vi "生成校准记录.vi"(0 "标液一":cluster{"标准值":dbl, "检测值":dbl, "原始值":dbl} caption="标液一：" {"原始值" format="%#.6f"; "检测值" format="%#.6f"; "标准值" format="%#.6f"}, 1 "校准参数":u16(ring) caption="校准参数：" items=["pH", "DO", "浊度", "电导率", "叶绿素a", "藻密度", "ORP", "COD", "DO2", "氯化物", "氨氮", "水中油"], 2 "校准方式":u16(ring) caption="校准方式：" items=["单点校准", "两点校准", "三点校准"], 3 "校准记录":refnum<vi>, 5 "标液二":cluster{"标准值":dbl, "检测值":dbl, "原始值":dbl} caption="标液二：" {"原始值" format="%#.6f"; "检测值" format="%#.6f"; "标准值" format="%#.6f"}, 7 "标液三":cluster{"标准值":dbl, "检测值":dbl, "原始值":dbl} caption="标液三：" {"原始值" format="%#.6f"; "检测值" format="%#.6f"; "标准值" format="%#.6f"}, 9 "当前温度":dbl caption="当前温度：" format="%.2f ℃", 11 "error in (no error)":errorcluster caption="错误输入（无错误）", 12 "序列号":string caption="序列号：", 13 "K":dbl=25.0 caption="电极系数：" format="%#_6f", 14 "B":dbl=25.0 caption="电极零点：" format="%#_6f") -> (4 "校准记录":string="校准记录\n---------------------------------------------\n序列号：\n温度值：\n标准值：\n检测值：\n原始值：\n校准时间：", 15 "error out":errorcluster caption="错误输出")   [LabVIEW 2022 SP3, in "斯坦道多参数.lvlib"]
uses:
  <vilib>/Utility/miscctls.llb/LVFontTypeDef.ctl
panel:
  in  "选项卡控件":enum32{"选项卡 1"}(tab)
  # "检测值"
  # "原始值"
  # "标准值"
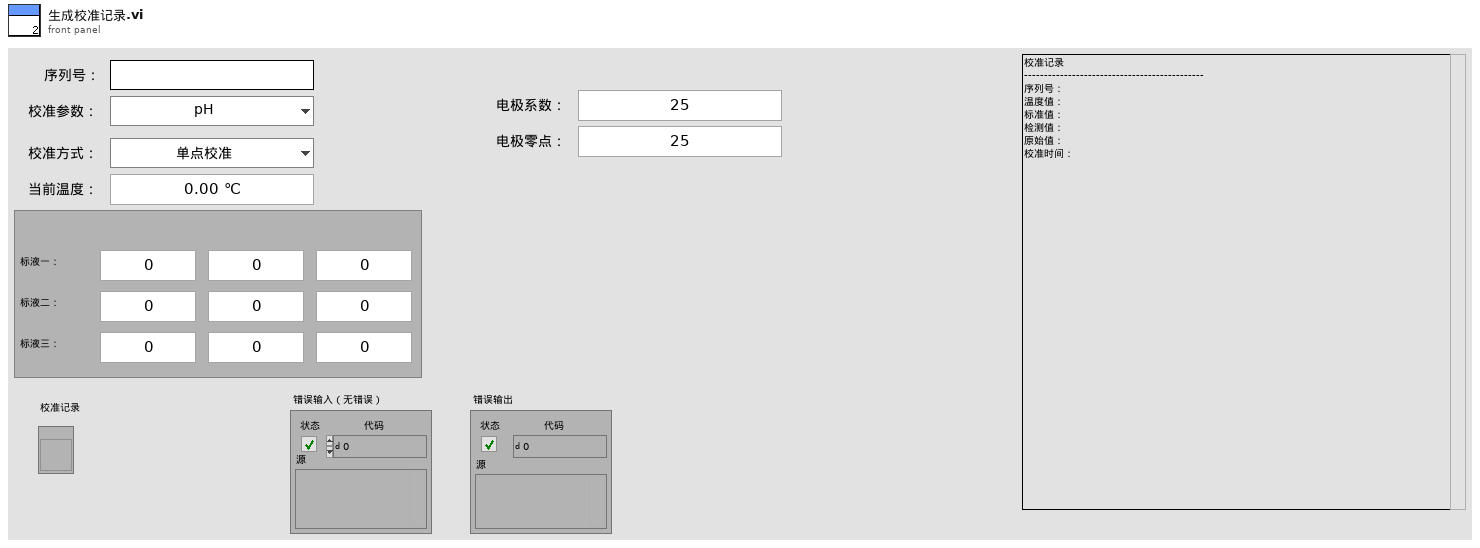
[diagram p1: front panel]
types:
  T1 = typedef "LVFontTypeDef.ctl" = cluster{"Font Name":string, "Size":u16, "Bold":bool, "Italic":bool, "Underline":bool, "Strikeout":bool, "Color":u32}
  T2 = typedef "斯坦道多参数.lvlib/探头类型.ctl" = enum16{"禹山", "国弘", "纳清", "STD"}
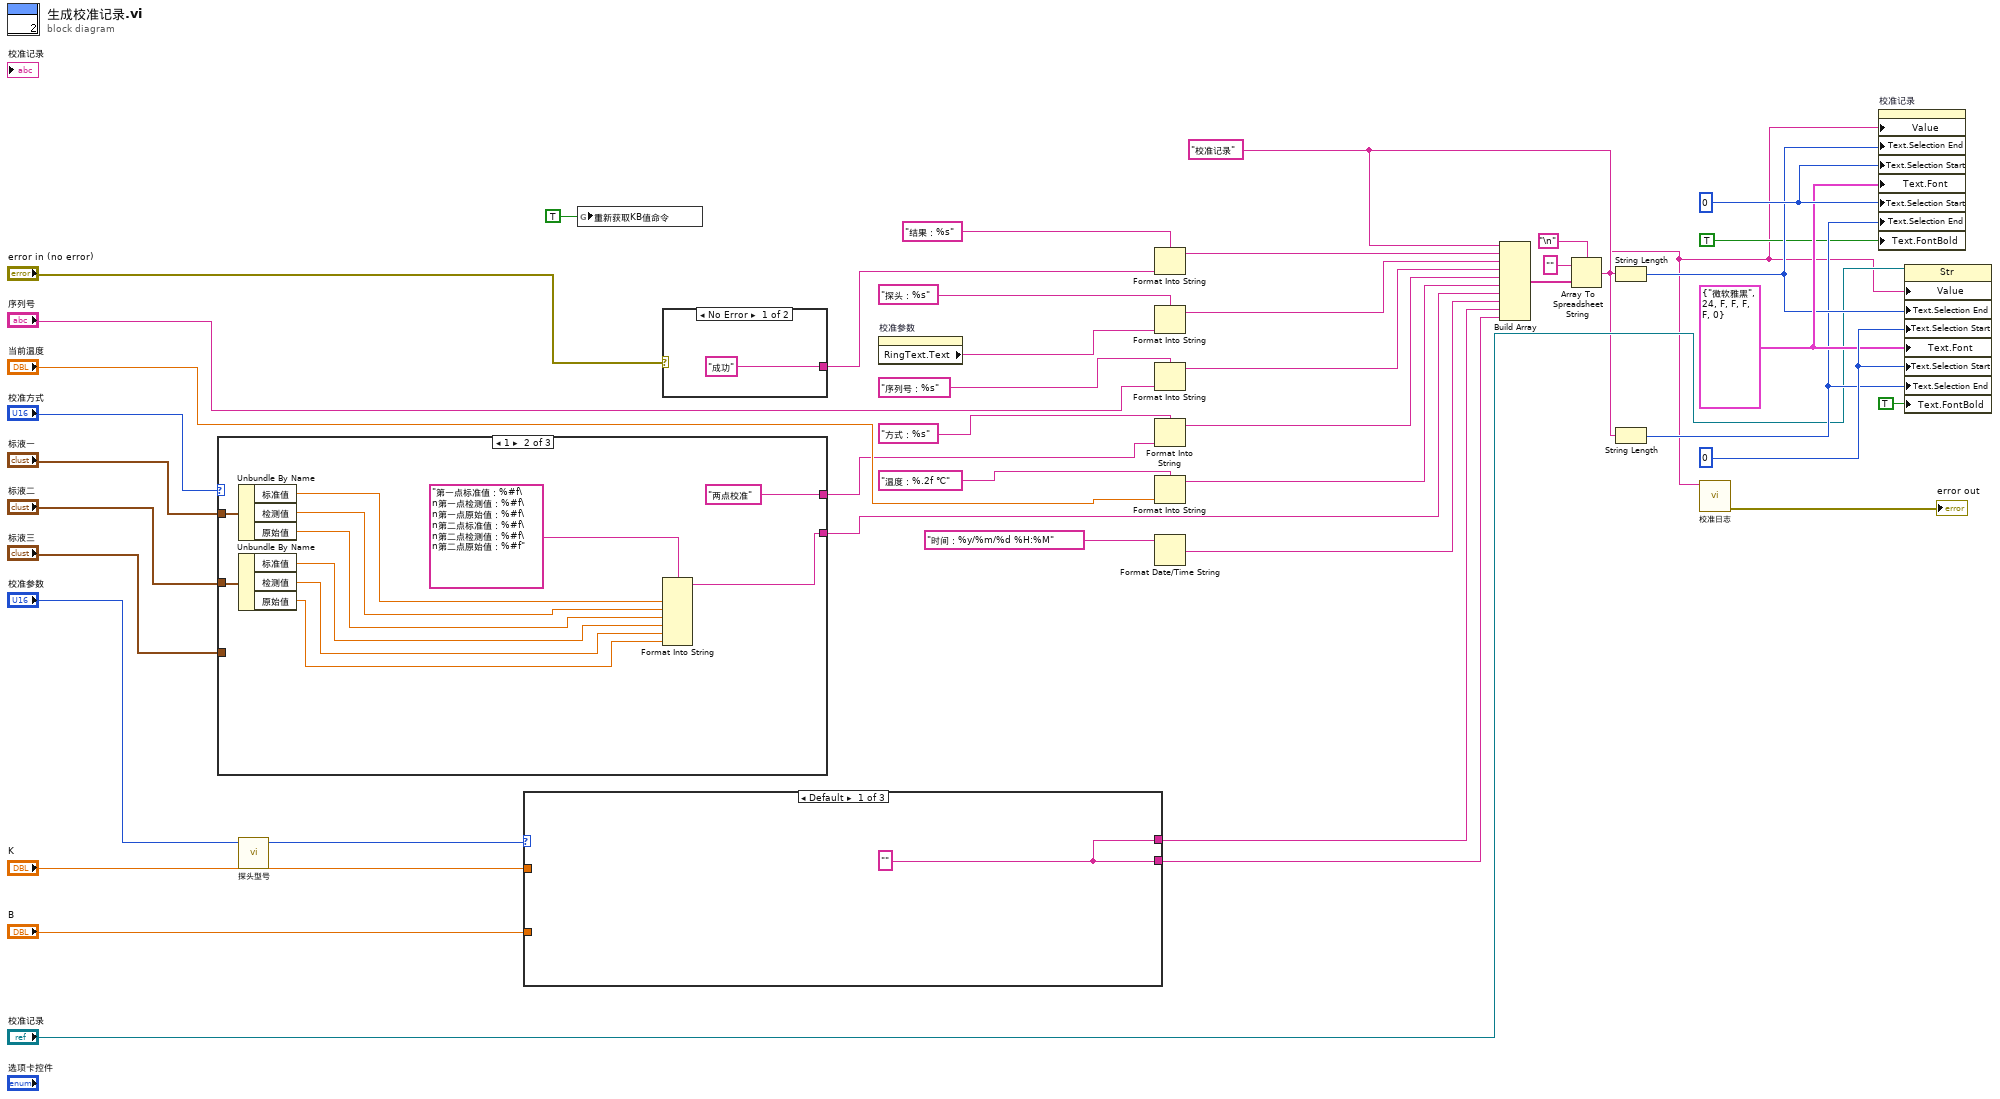
[diagram p0: block diagram]
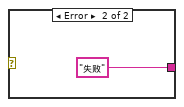
[diagram p2: hidden frame]
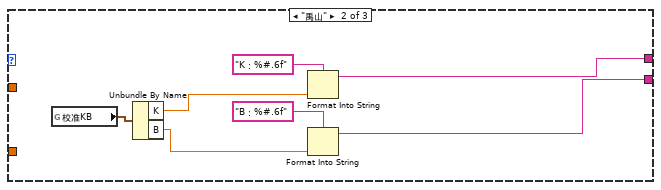
[diagram p3: hidden frame]
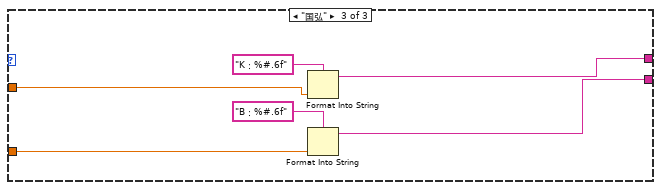
[diagram p4: hidden frame]
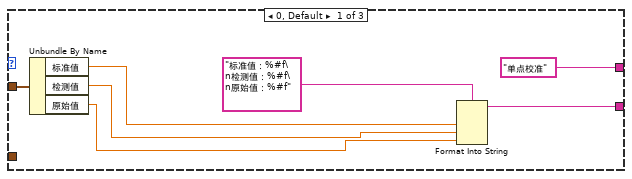
[diagram p5: hidden frame]
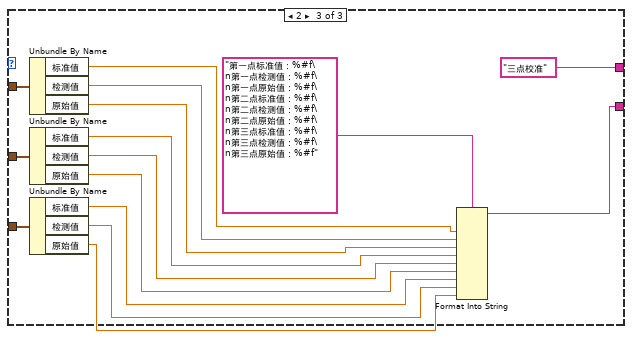
[diagram p6: hidden frame]
diagram:
  w20 = u32 0 ("文本.选择区域:起始")
  w22 = u32 0 ("文本.选择区域:起始")
  w19 = T1 {"Font Name"="微软雅黑", "Size"=24, "Bold"=FALSE, "Italic"=FALSE, "Underline"=FALSE, "Strikeout"=FALSE, "Color"=0} ("文本.字体")
  w8 = "校准记录"
  n1 = case shown="1" "校准方式" {
    tunnel: ["单点校准" "两点校准" "三点校准"] -> w38
    tunnel: [w49 w60 w67] -> w28
    tunnel: "标液一" -> [w48 w59 w68]
    tunnel: "标液二" -> [_ w55 w69]
    tunnel: "标液三" -> [_ _ w66]
    frame 0, Default {
      n2 = Unbundle By Name(w48) -> ("标准值"=w47:dbl, "检测值"=w46:dbl, "原始值"=w45:dbl)
      n3 = Format Into String(format string="标准值：%#f\n检测值：%#f\n原始值：%#f", w47, w46, w45) -> (resulting string=w49:string)  [unwired: 2 in, 1 out]
    }
    frame 1 {
      n4 = Unbundle By Name(w59) -> ("标准值"=w56:dbl, "检测值"=w57:dbl, "原始值"=w58:dbl)
      n5 = Unbundle By Name(w55) -> ("标准值"=w54:dbl, "检测值"=w53:dbl, "原始值"=w52:dbl)
      n6 = Format Into String(format string="第一点标准值：%#f\n第一点检测值：%#f\n第一点原始值：%#f\n第二点标准值：%#f\n第二点检测值：%#f\n第二点原始值：%#f", w56, w57, w58, w54, w53, w52) -> (resulting string=w60:string)  [unwired: 2 in, 1 out]
    }
    frame 2 {
      n7 = Unbundle By Name(w68) -> ("标准值"=w73:dbl, "检测值"=w74:dbl, "原始值"=w75:dbl)
      n8 = Unbundle By Name(w69) -> ("标准值"=w72:dbl, "检测值"=w71:dbl, "原始值"=w70:dbl)
      n9 = Unbundle By Name(w66) -> ("标准值"=w65:dbl, "检测值"=w64:dbl, "原始值"=w63:dbl)
      n10 = Format Into String(format string="第一点标准值：%#f\n第一点检测值：%#f\n第一点原始值：%#f\n第二点标准值：%#f\n第二点检测值：%#f\n第二点原始值：%#f\n第三点标准值：%#f\n第三点检测值：%#f\n第三点原始值：%#f", w73, w74, w75, w72, w71, w70, w65, w64, w63) -> (resulting string=w67:string)  [unwired: 2 in, 1 out]
    }
  }
  n11 = call "探头型号.vi"("校准参数"="校准参数") -> ("探头型号"=w13:T2)  [unwired: 8 in, 2 out]
  n12 = case shown="Default" w13 {
    tunnel: "K" -> [_ _ w91]
    tunnel: "B" -> [_ _ w88]
    tunnel: [w78 w83 w87] -> w10
    tunnel: [w78 w82 w86] -> w9
    frame Default {
      w78 = ""
    }
    frame "禹山" {
      n13 = global read "多参数全局变量.vi" "校准KB"() -> (w81:cluster{"K":sgl, "B":sgl})
      n14 = Unbundle By Name(w81) -> ("K"=w80:sgl, "B"=w79:sgl)
      n15 = Format Into String(format string="K：%#.6f" ("格式字符串"), w80) -> (resulting string=w83:string)  [unwired: 2 in, 1 out]
      n16 = Format Into String(format string="B：%#.6f" ("格式字符串"), w79) -> (resulting string=w82:string)  [unwired: 2 in, 1 out]
    }
    frame "国弘" {
      n17 = Format Into String(format string="K：%#.6f" ("格式字符串"), w91) -> (resulting string=w87:string)  [unwired: 2 in, 1 out]
      n18 = Format Into String(format string="B：%#.6f" ("格式字符串"), w88) -> (resulting string=w86:string)  [unwired: 2 in, 1 out]
    }
  }
  n19 = global write "多参数全局变量.vi" "重新获取KB值命令"(TRUE ("重新获取KB值命令")) -> ()
  n20 = case shown="No Error" "error in (no error)" {
    tunnel: ["成功" "失败"] -> w5
    frame No Error {
    }
    frame Error {
    }
  }
  n21 = property on="校准参数" class="Ring (strict)"() -> ("RingText.Text"=w36:string)  [unwired: 2 in, 2 out]
  n22 = Format Into String(format string="结果：%s" ("格式字符串"), w5) -> (resulting string=w6:string)  [unwired: 2 in, 1 out]
  n23 = Format Into String(format string="探头：%s", w36) -> (resulting string=w32:string)  [unwired: 2 in, 1 out]
  n24 = Format Into String(format string="序列号：%s", "序列号") -> (resulting string=w31:string)  [unwired: 2 in, 1 out]
  n25 = Format Into String(format string="方式：%s", w38) -> (resulting string=w30:string)  [unwired: 2 in, 1 out]
  n26 = Format Into String(format string="温度：%.2f ℃", "当前温度") -> (resulting string=w29:string)  [unwired: 2 in, 1 out]
  n27 = Format Date/Time String(time format string (%c)="时间：%y/%m/%d %H:%M" ("时间格式字符串(%c)")) -> (date/time string=w23:string)  [unwired: 2 in]
  n28 = Build Array(w8, w6, w32, w31, w30, w29, w28, w23, w10, w9) -> (w27:string[])
  n29 = Array To Spreadsheet String(delimiter (Tab)="\n", array=w27, 3:"" ("格式字符串")) -> (spreadsheet string=w3:string)
  n30 = String Length(string=w3) -> (length=w18:i32)
  n31 = String Length(string=w8) -> (length=w17:i32)
  n32 = call "校准日志.vi"("日志信息"=w3) -> ("error out"=→"error out":errorcluster)  [unwired: 10 in]
  n33 = property on="校准记录" class="Str"("Value"=w3, "Text.Selection End"=w18, "Text.Selection Start"=w20, "Text.Font"=w19, "Text.Selection Start"=w20, "Text.Selection End"=w17, "Text.FontBold"=TRUE ("文本.字体:粗体")) -> ()  [unwired: 2 in, 2 out]
  n34 = property class="Str"(reference="校准记录", "Value"=w3, "Text.Selection End"=w18, "Text.Selection Start"=w22, "Text.Font"=w19, "Text.Selection Start"=w22, "Text.Selection End"=w17, "Text.FontBold"=TRUE ("文本.字体:粗体")) -> ()  [unwired: 1 in, 2 out]
